vi "Add Exported VI.vi"(8 "error in (no error)":errorcluster, 10 "ProjectItem Refnum":refnum<vi>, 11 "DLL in":refnum<class "NI_AB_API_DLL.lvclass">) -> (0 "error out":errorcluster, 3 "DLL out":refnum<class "NI_AB_API_DLL.lvclass">)   [LabVIEW 2020, in "NI_AB_API_DLL.lvclass"]
uses:
  <vilib>/AppBuilder/AB_API/DLL/NI_AB_API_DLL.lvclass
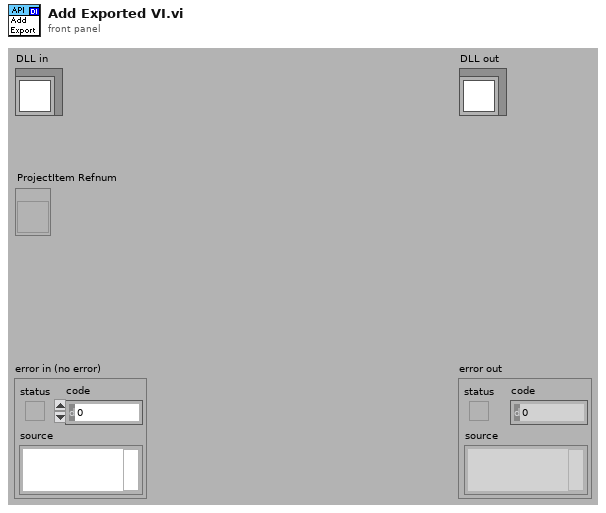
[diagram p1: front panel]
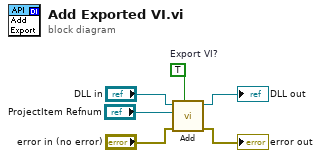
[diagram p0: block diagram]
diagram:
  w4 = TRUE  # Export VI?
  n1 = call <vilib>:"Add.vi"("Export VI?"=w4, "error in (no error)"="error in (no error)", "ProjectItem Refnum"="ProjectItem Refnum", "DLL in"="DLL in") -> ("error out"=→"error out":errorcluster, "DLL out"=→"DLL out":refnum<class "NI_AB_API_DLL.lvclass">)  [unwired: 6 in]
